vi "Load Display Settings.vi"(8 "error in (no error)":errorcluster, 11 "HIJ IMAQdx Display in":refnum<class "HIJ IMAQdx Display.lvclass">) -> (0 "error out":errorcluster, 3 "HIJ IMAQdx Display out":refnum<class "HIJ IMAQdx Display.lvclass">)   [LabVIEW 2020, in "HIJ IMAQdx Display.lvlib" / "HIJ IMAQdx Display.lvclass"]
doc: "Lade Anzeigeeinstellungen. Typischer Weise sind sie von der Kamera abhängig. Also wird aus dem Konfigpfad die Datei <Camera name>.xdcnf geladen."
uses:
  HIJ IMAQdx Display.lvclass
  HIJ IMAQdx Display.lvclass/HIJ IMAQdx Display.ctl
  Utility/POLARIS Vision utility.lvlib
  Analyze/Analyze Parameter/Analyze Parameter Target Point/Target Point.lvclass
  HIJ Vision Display/HIJ Vision Display/HIJ Vision Display.lvclass
  <vilib>/ActorFramework/Actor/Actor.lvclass
  Application Base Actors/HIJ Vision Application/HIJ Vision Application Messages/Set Parameter Msg/Set Parameter Msg.lvclass
  C:/Users/AlexK/work/LabVIEW Programme/POLARIS-AS-3-Cams/Submodules/HIJ Vision/Display Actors/HIJ Vision Display/HIJ Vision Display/HIJ Vision Display.lvclass
  C:/Users/AlexK/work/LabVIEW Programme/POLARIS-AS-3-Cams/Submodules/Viewable Actor/ViewableActor/ViewableActor.lvclass
  C:/Program Files (x86)/National Instruments/LabVIEW 2020/vi.lib/ActorFramework/Actor/Actor.lvclass
  C:/Users/AlexK/work/LabVIEW Programme/POLARIS-AS-3-Cams/Submodules/HIJ Vision/Analyze/Analyze Actor/IAnalysis/IAnalysis.lvclass
  C:/Users/AlexK/work/LabVIEW Programme/POLARIS-AS-3-Cams/Submodules/HIJ Vision/Camera Actors/Camera Actor/ICamera/ICamera.lvclass
  C:/Users/AlexK/work/LabVIEW Programme/POLARIS-AS-3-Cams/Submodules/HIJ Vision/Display Actors/HIJ IMAQdx Display/AF IMAQ Display/HIJ IMAQdx Display.lvclass
  C:/Users/AlexK/work/LabVIEW Programme/POLARIS-AS-3-Cams/Submodules/HIJ Vision/Analyze/Analyze Parameter/Analyze Parameter Base/Analyze Parameter Base.lvclass
  C:/Users/AlexK/work/LabVIEW Programme/POLARIS-AS-3-Cams/Submodules/HIJ Vision/Analyze/Analyze Parameter/Analyze Parameter Target Point/Target Point.lvclass
  HIJ Vision Display/HIJ Vision Display/Named ROI.ctl
  HIJ Vision Display/HIJ Vision Display/DisplaySettings.ctl
panel:
  in  "ROI":T1 {"Contours"."Type" items=["No Selection", "Point", "Line", "Rectangle", "Oval", "Polygon", "Freehand Region", "Annulus", "Unused2", "Unused3", "Broken Line", "Freehand Line", "Rotated Rectangle"]}
  in  "Display settings":T2
  in  "Saved ROIs":T3[](array[typedef])
  in  "Image Center":cluster{"X":u32, "Y":u32}
  in  "Zoom":cluster{"X":i32, "Y":i32}
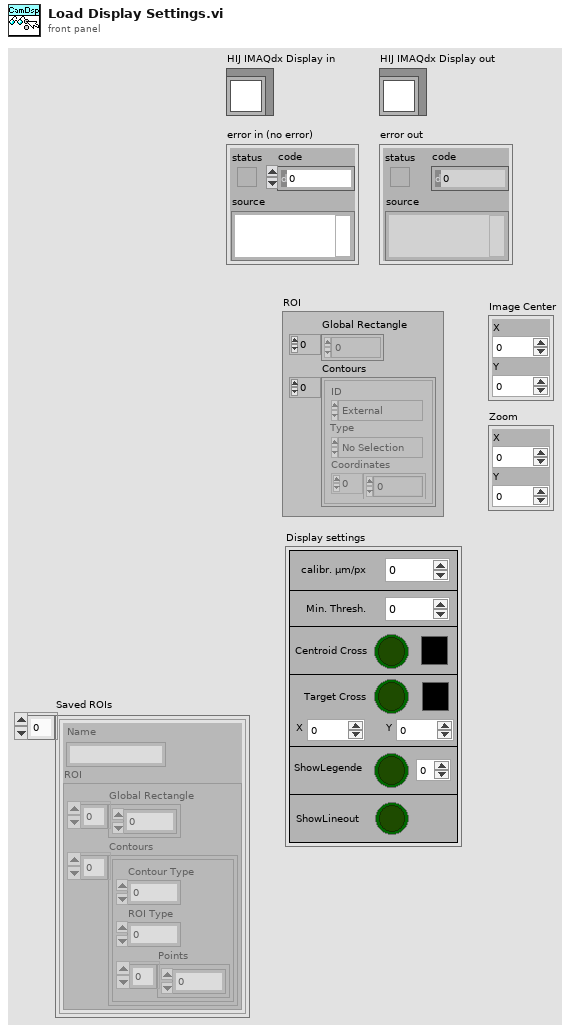
[diagram p1: front panel]
types:
  T1 = typedef "ROI Descriptor" = cluster{"Global Rectangle":i32[], "Contours":cluster{"ID":enum32{"External", "Internal"}, "Type":u32, "Coordinates":i32[]}[]}
  T2 = typedef "HIJ Vision Display.lvlib/HIJ Vision Display.lvclass/DisplaySettings.ctl" = cluster{"Min. Thresh.":sgl, "X":dbl, "Y":dbl, "ShowLineout":bool, "ScaleParts":i32, "ShowLegende":bool, "Target Cross":bool, "Centroid Cross":bool, "Target color":u32, "Centroid color":u32, "calibr. µm/px":sgl[unit]}
  T3 = typedef "HIJ Vision Display.lvlib/HIJ Vision Display.lvclass/Named ROI.ctl" = cluster{"ROI":cluster{"Global Rectangle":i32[], "Contours":cluster{"Contour Type":u32, "ROI Type":u32, "Points":i32[]}[]}, "Name":string}
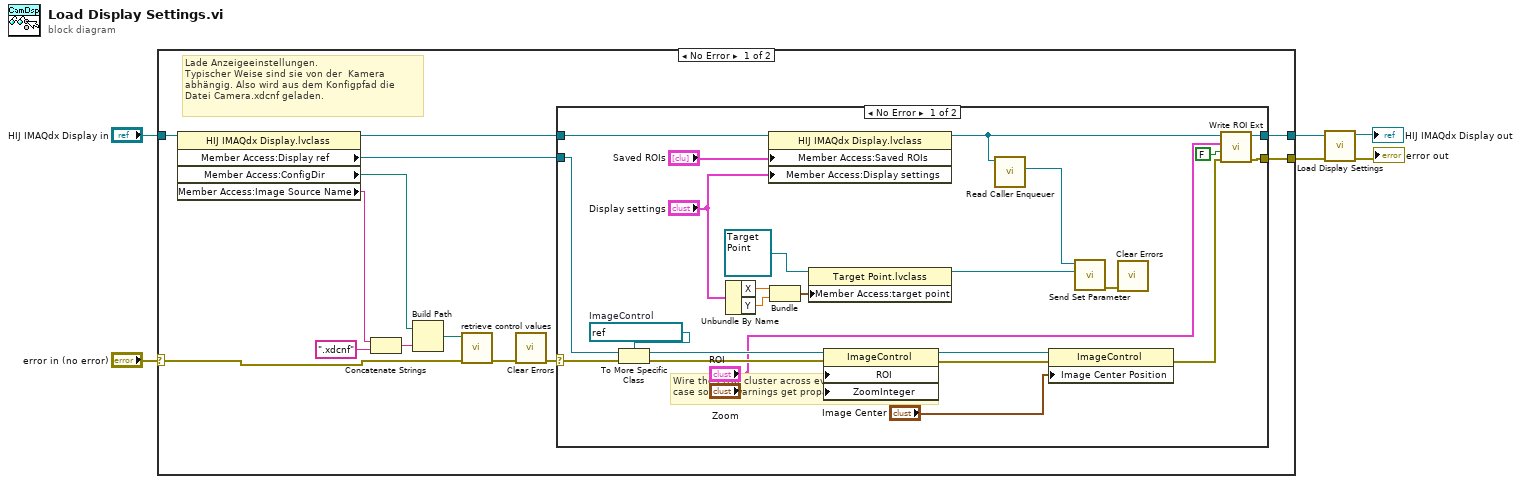
[diagram p0: block diagram]
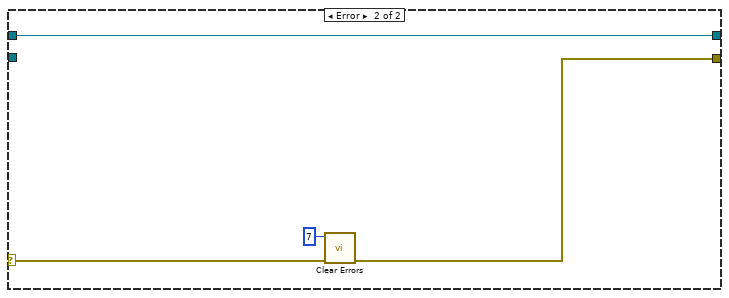
[diagram p2: hidden frame]
diagram:
  n1 = case shown="No Error" "error in (no error)" {
    selector: "error in (no error)" -> [w13 w50]
    tunnel: [w10 w50] -> w2
    tunnel: [w14 w49] -> w4
    tunnel: "HIJ IMAQdx Display in" -> [w9 w49]
    frame No Error {
      # "Lade Anzeigeeinstellungen.\nTypischer Weise sind sie von der  Kamera\nabhängig. Also wird aus dem Konfigpfad die \nDatei Camera.xdcnf geladen."
      # "Wire the error cluster across even in the \"No Error\"\ncase so that warnings get propagated."
      n2 = property class="HIJ IMAQdx Display.lvclass"(reference=w9) -> (reference out=w12:refnum<class "HIJ IMAQdx Display.lvclass">, "Member Access:Display ref"=w11:refnum<vi>, "Member Access:ConfigDir"=w7:path, "Member Access:Image Source Name"=w8:string)  [unwired: 1 in, 1 out]
      n3 = Concatenate Strings(w8, ".xdcnf" ("string")) -> (w17:string)
      n4 = Build Path(base path=w7, name or relative path=w17) -> (appended path=w15:path)
      n5 = call "retrieve control values.vi"("error in (no error)"=w13, "path"=w15) -> ("error out"=w16:errorcluster)  [unwired: 8 in, 1 out]
      n6 = call <vilib>:"Clear Errors.vi"("error in (no error)"=w16) -> ("error out"=w19:errorcluster)  [unwired: 5 in, 1 out]
      n7 = case shown="No Error" w19 {
        selector: w19 -> [w41 w48]
        tunnel: [w23 w46] -> w10
        tunnel: [w25 w47] -> w14
        tunnel: w12 -> [w26 w47]
        tunnel: w11 -> [w39 _]
        frame No Error {
          w38 = refnum<vi> refnum  # ImageControl
          n8 = To More Specific Class(target class=w38, reference=w39, error in=w41) -> (specific class reference=w42:refnum<vi>, error out=w43:errorcluster)
          n9 = Unbundle By Name("Display settings") -> ("X"=w32:dbl, "Y"=w31:dbl)
          n10 = property class="HIJ IMAQdx Display.lvclass"(reference=w26, "Member Access:Saved ROIs"="Saved ROIs", "Member Access:Display settings"="Display settings") -> (reference out=w21:refnum<class "HIJ IMAQdx Display.lvclass">)  [unwired: 1 in, 1 out]
          n11 = Bundle("X"=w32, "Y"=w31) -> (w30:cluster{"X":dbl, "Y":dbl})  [unwired: 1 in]
          n12 = property class="Target Point.lvclass"(reference=refnum<class "Target Point.lvclass"> refnum ("Target Point.lvclass"), "Member Access:target point"=w30) -> (reference out=w29:refnum<class "Target Point.lvclass">)  [unwired: 1 in, 1 out]
          n13 = property class="ImageControl"(reference=w42, error in=w43, "ROI"="ROI", "ZoomInteger"="Zoom") -> (reference out=w35:refnum<vi>, error out=w36:errorcluster)
          n14 = call <vilib>:"Read Caller Enqueuer.vi"("Actor"=w21) -> ("Caller Enqueuer"=w20:refnum<class "Message Enqueuer.lvclass">)  [unwired: 10 in]
          n15 = property class="ImageControl"(reference=w35, error in=w36, "Image Center Position"="Image Center") -> (error out=w24:errorcluster)  [unwired: 1 out]
          n16 = call "Send Set Parameter.vi"("Parameter"=w29, "Message Enqueuer"=w20) -> ("error out"=w28:errorcluster)  [unwired: 8 in, 1 out]
          n17 = call <vilib>:"Clear Errors.vi"("error in (no error)"=w28) -> ()  [unwired: 5 in, 2 out]
          n18 = call "Write ROI Ext.vi"("error in (no error)"=w24, "Save to File"=FALSE, "ROI Descriptor"="ROI", "IMAQ Display in"=w21) -> ("error out"=w23:errorcluster, "IMAQ Display out"=w25:refnum<class "HIJ IMAQdx Display.lvclass">)  [unwired: 6 in]
        }
        frame Error {
          n19 = call <vilib>:"Clear Errors.vi"("error in (no error)"=w48, "specific error code to clear (0: all)"=7) -> ("error out"=w46:errorcluster)  [unwired: 4 in, 1 out]
        }
      }
    }
    frame Error {
    }
  }
  n20 = call-parent "Load Display Settings.vi"("error in (no error)"=w2, "AF IMAQ Display in"=w4) -> ("error out"=→"error out":errorcluster, "AF IMAQ Display out"=→"HIJ IMAQdx Display out":refnum<class "HIJ IMAQdx Display.lvclass">)  [unwired: 8 in]
